vi "MGI Natural Sort.vi"(10 "Unsorted Array":string[](array[string])) -> (1 "Pointers":i32[](array[numeric]), 2 "Sorted Array":string[](array[string]))   [LabVIEW 2016]
doc: "Sorts the string array by natural order. This means that something like \"T2\" will come before \"T10\". For Example:\n\nUsing the array: [\"T2\", \"T10\", \"T1\"]\nBuilt in 1D Array Sort Results: [\"T1\", \"T10\", \"T2\"]\nNatural Sort Results: [\"T1\", \"T2\", \"T10\"]\n\nCopyright: MGI\nAuthored By: Derek Trepanier"
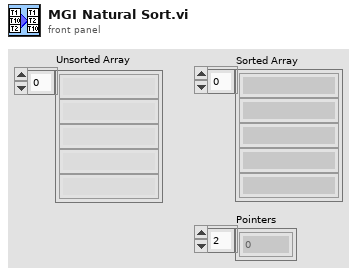
[diagram p1: front panel]
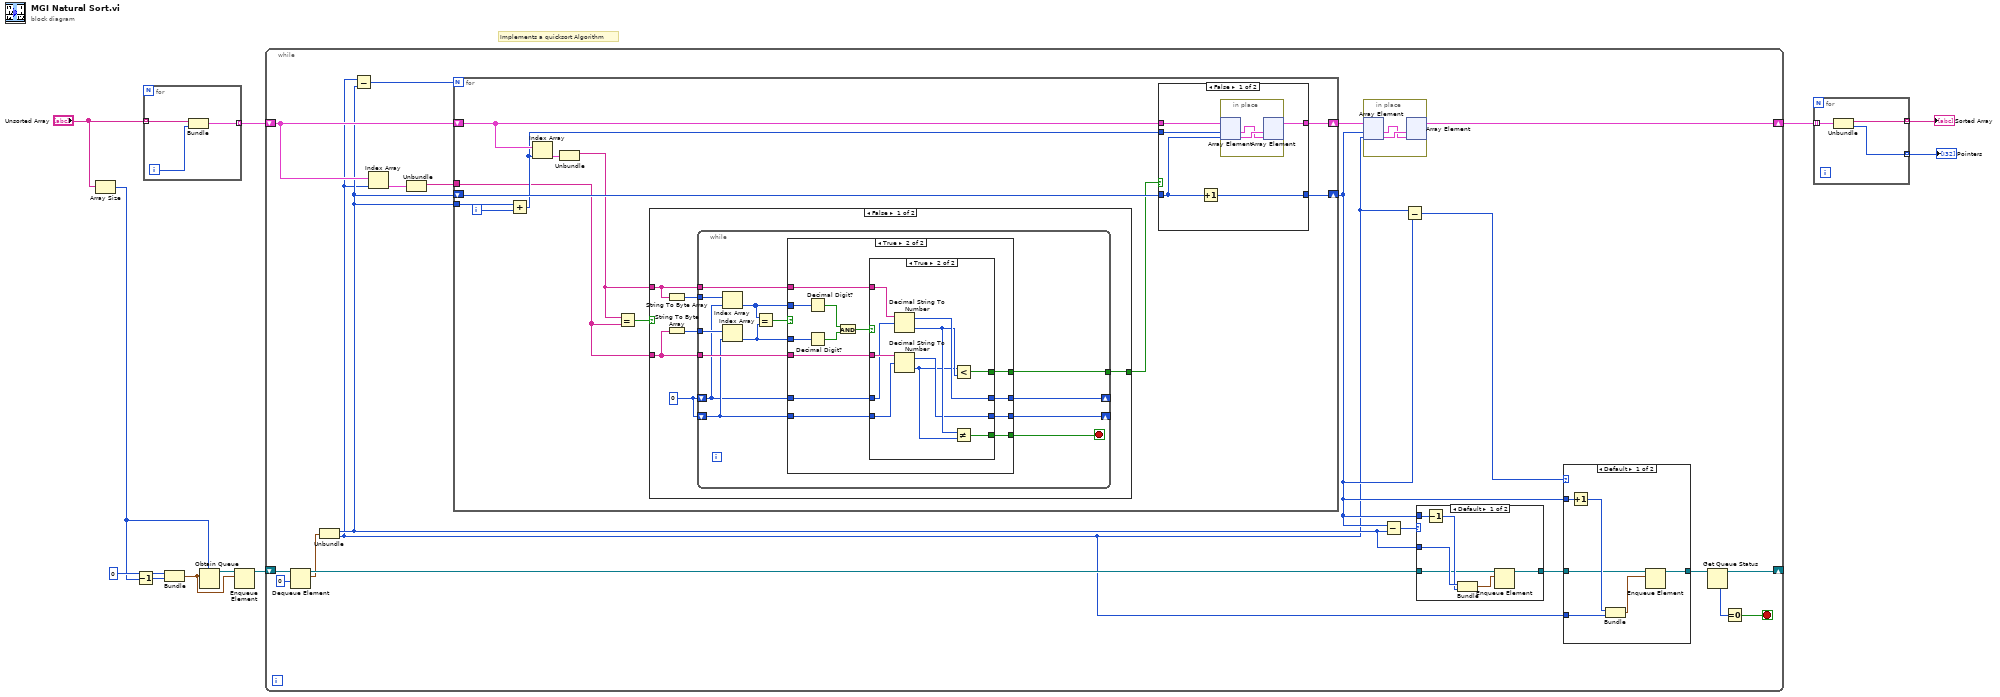
[diagram p0: block diagram]
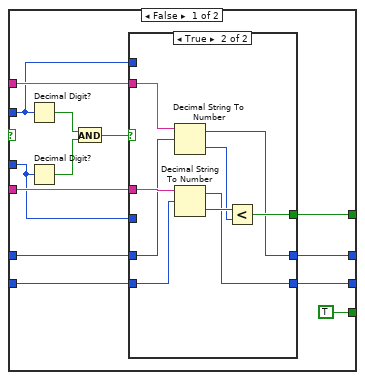
[diagram p4: hidden frame]
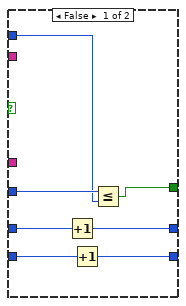
[diagram p5: hidden frame]
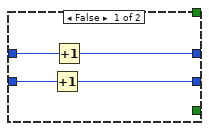
[diagram p6: hidden frame]
diagram:
  # "Implements a quicksort Algorithm"
  n1 = Array Size(array="Unsorted Array") -> (size(s)=w6:i32)
  n2 = Decrement(x=w6) -> (x-1=w10:i32)
  n3 = for {
    tunnel: "Unsorted Array" -> [w14] mode=indexing
    tunnel: [w12] -> w4 mode=indexing
    i -> [w13]
    n4 = Bundle("String"=w14, w13) -> (w12:cluster{"String":string, i32})  [unwired: 1 in]
  }
  n5 = Bundle("size(s)"=0, w10) -> (w7:cluster{"size(s)":i32, i32})  [unwired: 1 in]
  n6 = Obtain Queue(max queue size (-1, unlimited)=w6, element data type=w7) -> (queue out=w9:refnum<queue>)  [unwired: 3 in, 2 out]
  n7 = Enqueue Element(queue=w9, element=w7) -> (queue out=w8:refnum<queue>)  [unwired: 2 in, 2 out]
  n8 = while {
    shift-right: [w18] -> _
    shift-left: w8 -> [w34]
    shift-right: [w29] -> w3
    shift-left: w4 -> [w31]
    stop <- w16 stop-if-true
    n9 = Dequeue Element(queue=w34, timeout in ms (-1)=0) -> (queue out=w27:refnum<queue>, element=w21:cluster{"size(s)":i32, i32})  [unwired: 1 in, 2 out]
    n10 = Unbundle(w21) -> ("size(s)"=w26:i32, w22:i32)
    n11 = Subtract(x=w22, y=w26) -> (x-y=w33:i32)
    n12 = Index Array(array=w31, index=w22) -> (element=w32:cluster{"String":string, i32})
    n13 = Unbundle(w32) -> ("String"=w15:string)  [unwired: 1 out]
    n14 = for {
      N: w33 -> [_]
      shift-right: [w59] -> w30
      shift-left: w31 -> [w60]
      tunnel: w26 -> [w61]
      tunnel: w15 -> [w53]
      shift-right: [w57] -> w23
      shift-left: w26 -> [w58]
      i -> [w62]
      n15 = Add(x=w61, y=w62) -> (x+y=w56:i32)
      n16 = Index Array(array=w60, index=w56) -> (element=w54:cluster{"String":string, i32})
      n17 = Unbundle(w54) -> ("String"=w51:string)  [unwired: 1 out]
      n18 = Equal?(x=w51, y=w53) -> (x = y?=w52:bool)
      n19 = case shown="False" w52 {
        tunnel: w51 -> [w66 _]
        tunnel: w53 -> [w65 _]
        tunnel: [w64 _] -> w55
        frame False {
          w63 = 0
          n20 = String To Byte Array(string=w66) -> (unsigned byte array=w68:u8[])
          n21 = String To Byte Array(string=w65) -> (unsigned byte array=w67:u8[])
          n22 = while {
            tunnel: w68 -> [w76]
            tunnel: w67 -> [w74]
            tunnel: w65 -> [w79]
            tunnel: w66 -> [w80]
            tunnel: [w78] -> w64
            shift-right: [w70] -> _
            shift-left: w63 -> [w71]
            shift-right: [w69] -> _
            shift-left: w63 -> [w72]
            stop <- w77 stop-if-true
            n23 = Index Array(array=w76, index=w71) -> (element=w75:u8)
            n24 = Index Array(array=w74, index=w72) -> (element=w73:u8)
            n25 = Equal?(x=w75, y=w73) -> (x = y?=w81:bool)
            n26 = case shown="True" w81 {
              tunnel: w80 -> [w89 w118]
              tunnel: w79 -> [w88 w117]
              tunnel: w75 -> [w86 w121]
              tunnel: w73 -> [w85 w120]
              tunnel: [w91 w115] -> w78
              tunnel: [TRUE w111] -> w77
              tunnel: w71 -> [w87 w116]
              tunnel: w72 -> [w82 w114]
              tunnel: [w84 w113] -> w70
              tunnel: [w83 w112] -> w69
              frame False {
                n27 = Decimal Digit?(1:w86) -> (0:w92:bool)
                n28 = Decimal Digit?(1:w85) -> (0:w93:bool)
                n29 = And(x=w92, y=w93) -> (x .and. y?=w94:bool)
                n30 = case shown="True" w94 {
                  tunnel: [w99 w105] -> w91
                  tunnel: w89 -> [_ w110]
                  tunnel: w88 -> [_ w109]
                  tunnel: w87 -> [w98 w108]
                  tunnel: w86 -> [w100 _]
                  tunnel: w85 -> [w101 _]
                  tunnel: [w95 w104] -> w84
                  tunnel: [w96 w103] -> w83
                  tunnel: w82 -> [w97 w102]
                  frame False {
                    n31 = Increment(x=w98) -> (x+1=w95:i32)
                    n32 = Increment(x=w97) -> (x+1=w96:i32)
                    n33 = Less Or Equal?(x=w101, y=w100) -> (x <= y?=w99:bool)
                  }
                  frame True {
                    n34 = Decimal String To Number(string=w110, offset=w108) -> (offset past number=w104:i32, number=w106:i32)  [unwired: 1 in]
                    n35 = Decimal String To Number(string=w109, offset=w102) -> (offset past number=w103:i32, number=w107:i32)  [unwired: 1 in]
                    n36 = Less?(x=w107, y=w106) -> (x < y?=w105:bool)
                  }
                }
              }
              frame True {
                n37 = Decimal Digit?(1:w121) -> (0:w122:bool)
                n38 = Decimal Digit?(1:w120) -> (0:w123:bool)
                n39 = And(x=w122, y=w123) -> (x .and. y?=w119:bool)
                n40 = case shown="True" w119 {
                  tunnel: w118 -> [_ w137]
                  tunnel: w117 -> [_ w136]
                  tunnel: w116 -> [w127 w135]
                  tunnel: [_ w134] -> w115
                  tunnel: w114 -> [w126 w133]
                  tunnel: [w125 w132] -> w113
                  tunnel: [w124 w130] -> w112
                  tunnel: [_ w129] -> w111
                  frame False {
                    n41 = Increment(x=w126) -> (x+1=w124:i32)
                    n42 = Increment(x=w127) -> (x+1=w125:i32)
                  }
                  frame True {
                    n43 = Decimal String To Number(string=w137, offset=w135) -> (offset past number=w132:i32, number=w131:i32)  [unwired: 1 in]
                    n44 = Decimal String To Number(string=w136, offset=w133) -> (offset past number=w130:i32, number=w128:i32)  [unwired: 1 in]
                    n45 = Not Equal?(x=w131, y=w128) -> (x != y?=w129:bool)
                    n46 = Less?(x=w128, y=w131) -> (x < y?=w134:bool)
                  }
                }
              }
            }
          }
        }
        frame True {
        }
      }
      n47 = case shown="False" w55 {
        tunnel: w60 -> [w142 w146]
        tunnel: [w141 w146] -> w59
        tunnel: w58 -> [w140 w145]
        tunnel: [w138 w145] -> w57
        tunnel: w56 -> [w139 _]
        frame False {
          n48 = Increment(x=w140) -> (x+1=w138:i32)
          n49 = in-place {
            n50 = in-place-array #1(w142, w139, w140) -> (w143:cluster{"String":string, i32}, w144:cluster{"String":string, i32})
            n51 = in-place-array #1(w144, w143) -> (w141:cluster{"String":string, i32}[])  [unwired: 2 out]
          }
        }
        frame True {
        }
      }
    }
    n52 = in-place {
      n53 = in-place-array #2(w30, w23, w22) -> (w49:cluster{"String":string, i32}, w50:cluster{"String":string, i32})
      n54 = in-place-array #2(w50, w49) -> (w29:cluster{"String":string, i32}[])  [unwired: 2 out]
    }
    n55 = Subtract(x=w23, y=w26) -> (x-y=w28:i32)
    n56 = Subtract(x=w22, y=w23) -> (x-y=w24:i32)
    n57 = case shown="Default" w28 {
      tunnel: w27 -> [w44 w48]
      tunnel: [w43 w48] -> w25
      tunnel: w26 -> [w47 _]
      tunnel: w23 -> [w46 _]
      frame Default {
        n58 = Decrement(x=w46) -> (x-1=w45:i32)
        n59 = Bundle("size(s)"=w47, w45) -> (w42:cluster{"size(s)":i32, i32})  [unwired: 1 in]
        n60 = Enqueue Element(queue=w44, element=w42) -> (queue out=w43:refnum<queue>)  [unwired: 2 in, 2 out]
      }
      frame ..1 {
      }
    }
    n61 = case shown="Default" w24 {
      tunnel: w25 -> [w37 w41]
      tunnel: [w36 w41] -> w19
      tunnel: w23 -> [w40 _]
      tunnel: w22 -> [w38 _]
      frame Default {
        n62 = Increment(x=w40) -> (x+1=w39:i32)
        n63 = Bundle(w39, w38) -> (w35:cluster{i32, i32})  [unwired: 1 in]
        n64 = Enqueue Element(queue=w37, element=w35) -> (queue out=w36:refnum<queue>)  [unwired: 2 in, 2 out]
      }
      frame ..1 {
      }
    }
    n65 = Get Queue Status(queue=w19) -> (queue out=w18:refnum<queue>, # elements in queue=w17:i32)  [unwired: 2 in, 6 out]
    n66 = Equal To 0?(x=w17) -> (x = 0?=w16:bool)
  }
  n67 = for {
    tunnel: w3 -> [w149] mode=indexing
    tunnel: [w148] -> w2 mode=indexing
    tunnel: [w147] -> w1 mode=indexing
    n68 = Unbundle(w149) -> ("String"=w148:string, w147:i32)
  }
  "Sorted Array" <- w2
  "Pointers" <- w1
